vi "OpenShortDeembed_Framework.vi"() -> ()   [LabVIEW 2020]
uses:
  <vilib>/addons/HF Network Analysis/Support VIs/Read SnP File (SnP).vi
  <vilib>/addons/HF Network Analysis/NI_HFNetworkAnalysis.lvlib
panel:
  out "Snp Path Out":path
  in  "Comments":string
  in  "Short SnP File Path":path
  in  "Open SnP File Path":path
  out "Error Out":errorcluster
  in  "Error In":errorcluster
  in  "Non-DeEmbedded DUT SnP File Path":path
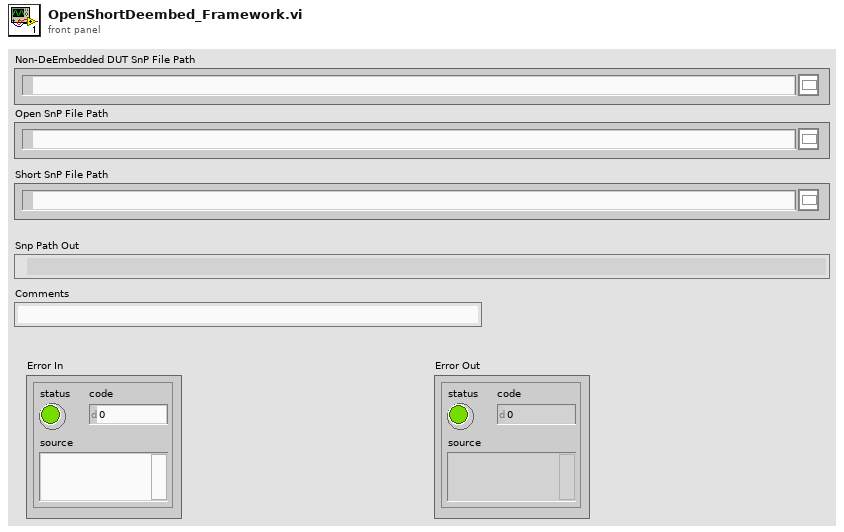
[diagram p1: front panel]
types:
  T1 = cluster{"Comments":string, "Ref Impedance":u16, "Trace Array":cluster{"Freq (Hz)":dbl, "S-parameter Array":cdb[][]}[]}
  T2 = cluster{"Freq (Hz)":dbl, "S-parameter Array":cdb[][]}[]
  T3 = cluster{"Freq (Hz)":dbl, "S-parameter Array":csg[][]}[]
  T4 = cluster{string, "Z0 (Ohm)":cdb, "Intrinsic DUT S-parameter Trace Array":cluster{"Freq (Hz)":dbl, "S-parameter Array":csg[][]}[]}
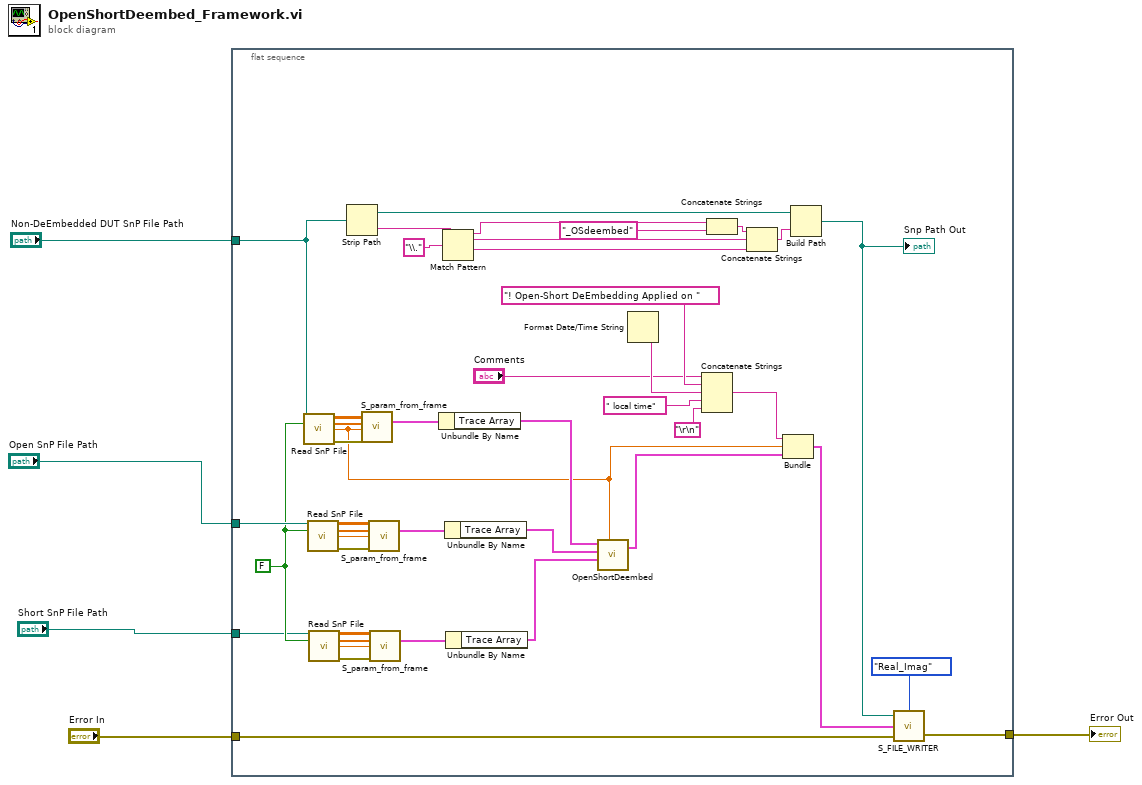
[diagram p0: block diagram]
diagram:
  n1 = flat-sequence {
    tunnel: "Non-DeEmbedded DUT SnP File Path" -> [w10]
    tunnel: "Open SnP File Path" -> [w39]
    tunnel: "Short SnP File Path" -> [w30]
    tunnel: "Error In" -> [w8]
    tunnel: [w7] -> w1
    frame #0 {
      w31 = FALSE ("Swap Ports (False)")
      n2 = call-poly <vilib>:"Read SnP File.vi"("SnP File Path"=w10, "Swap Ports (False)"=w31) -> ("S-parameters"=w47:cdb[][], "Frequencies (Hz)"=w46:dbl[], "Z0 (Ohm)"=w28:cdb, "Error Out"=w48:errorcluster)  [unwired: 10 in]
      n3 = call-poly <vilib>:"Read SnP File.vi"("SnP File Path"=w39, "Swap Ports (False)"=w31) -> ("S-parameters"=w43:cdb[][], "Frequencies (Hz)"=w42:dbl[], "Z0 (Ohm)"=w40:cdb, "Error Out"=w41:errorcluster)  [unwired: 10 in]
      n4 = call-poly <vilib>:"Read SnP File.vi"("SnP File Path"=w30, "Swap Ports (False)"=w31) -> ("S-parameters"=w32:cdb[][], "Frequencies (Hz)"=w33:dbl[], "Z0 (Ohm)"=w35:cdb, "Error Out"=w34:errorcluster)  [unwired: 10 in]
      n5 = Strip Path(path=w10) -> (stripped path=w19:path, name=w18:string)
      n6 = call "S_param_from_frame.VI"("S-parameter Array"=w47, "Frequencies (Hz)"=w46, "Ref Impedance"=w28, "error in (no error)"=w48) -> ("Data Output"=w45:T1)  [unwired: 10 in, 1 out]
      n7 = call "S_param_from_frame.VI"("S-parameter Array"=w43, "Frequencies (Hz)"=w42, "Ref Impedance"=w40, "error in (no error)"=w41) -> ("Data Output"=w38:T1)  [unwired: 10 in, 1 out]
      n8 = call "S_param_from_frame.VI"("S-parameter Array"=w32, "Frequencies (Hz)"=w33, "Ref Impedance"=w35, "error in (no error)"=w34) -> ("Data Output"=w36:T1)  [unwired: 10 in, 1 out]
      n9 = Unbundle By Name(w45) -> ("Trace Array"=w44:T2)
      n10 = Match Pattern(string=w18, regular expression="\\.") -> (before substring=w12:string, match substring=w14:string, after substring=w15:string)  [unwired: 1 in, 1 out]
      n11 = Unbundle By Name(w38) -> ("Trace Array"=w37:T2)
      n12 = Unbundle By Name(w36) -> ("Trace Array"=w29:T2)
      n13 = call "OpenShortDeembed.vi"("Extrinsic DUT S-parameter Trace Array"=w44, "Open S-parameter Trace Array"=w37, "Short S-parameter Trace Array"=w29, "Reference Impedance"=w28) -> ("Intrinsic DUT S-parameter Trace Array"=w27:T3)  [unwired: 1 in, 1 out]
      n14 = Format Date/Time String() -> (date/time string=w23:string)  [unwired: 3 in]
      n15 = Concatenate Strings("Comments", "! Open-Short DeEmbedding Applied on ", w23, " local time", "\r\n") -> (w21:string)
      n16 = Concatenate Strings(w12, "_OSdeembed") -> (w13:string)
      n17 = Concatenate Strings(w13, w14, w15) -> (w16:string)
      n18 = Bundle(w21, "Z0 (Ohm)"=w28, "Intrinsic DUT S-parameter Trace Array"=w27) -> (w26:T4)  [unwired: 1 in]
      n19 = Build Path(base path=w19, name or relative path=w16) -> (appended path=w9:path)
      "Snp Path Out" <- w9
      n20 = call "S_FILE_WRITER.VI"("Data Write Format"=enum16{"Real_Imag", "Mag_Angle", "dB_Angle"}."Real_Imag", "error in (no error)"=w8, "Data Input"=w26, "Input Path"=w9) -> ("error out"=w7:errorcluster)  [unwired: 1 out]
    }
  }
  "Error Out" <- w1
